vi "GEA2 FP ERDs.vi"(4 "2019 Inverter CMDs":T3[](array[typedef])=[{"ERD Number"=62218, "Data Type"=enum."string"}, {"ERD Number"=62229, "Data Type"=enum."string"}, {"ERD Number"=62224, "Data Type"=enum."string"}] {"ERD Number" format="%.0x"}, 6 "Inverter Address":T2={"Source"=240, "Destination"=63} {"Destination" format="%.0x"; "Source" format="%.0x"}, 8 "Error In":errorcluster, 10 "GEA2 Event Registration In":refnum<event-registration>, 11 ".NET Refnum in":refnum<k24>) -> (0 "Error Out":errorcluster, 1 "Data":string[][](array[string]), 2 "GEA2 Event Registration Out":refnum<event-registration>, 3 ".NET Refnum out":refnum<k24>, 5 "ERD Data Out":T1[](array[typedef]) {"ERD Number" format="%.0x"})   [LabVIEW 2016]
uses:
  type defs/ERD Read Data In.ctl
  type defs/Data Type.ctl
  type defs/Source_Destination.ctl
  C:/Technology Lab/NI-2010/Trunk/Utility/LabVIEW GEA2 Toolkit v1.0.0.0/Appliance.NET/GeaCommunication.dll
  Appliance.NET/GeaCommunication.dll
  type defs/Data Out.ctl
  type defs/ERD Read Data Out.ctl
  <vilib>/Utility/error.llb/whitespace.ctl
  library/GEA2_Toolkit.lvlib
panel:
  in  "#ERDs per message":i32=15
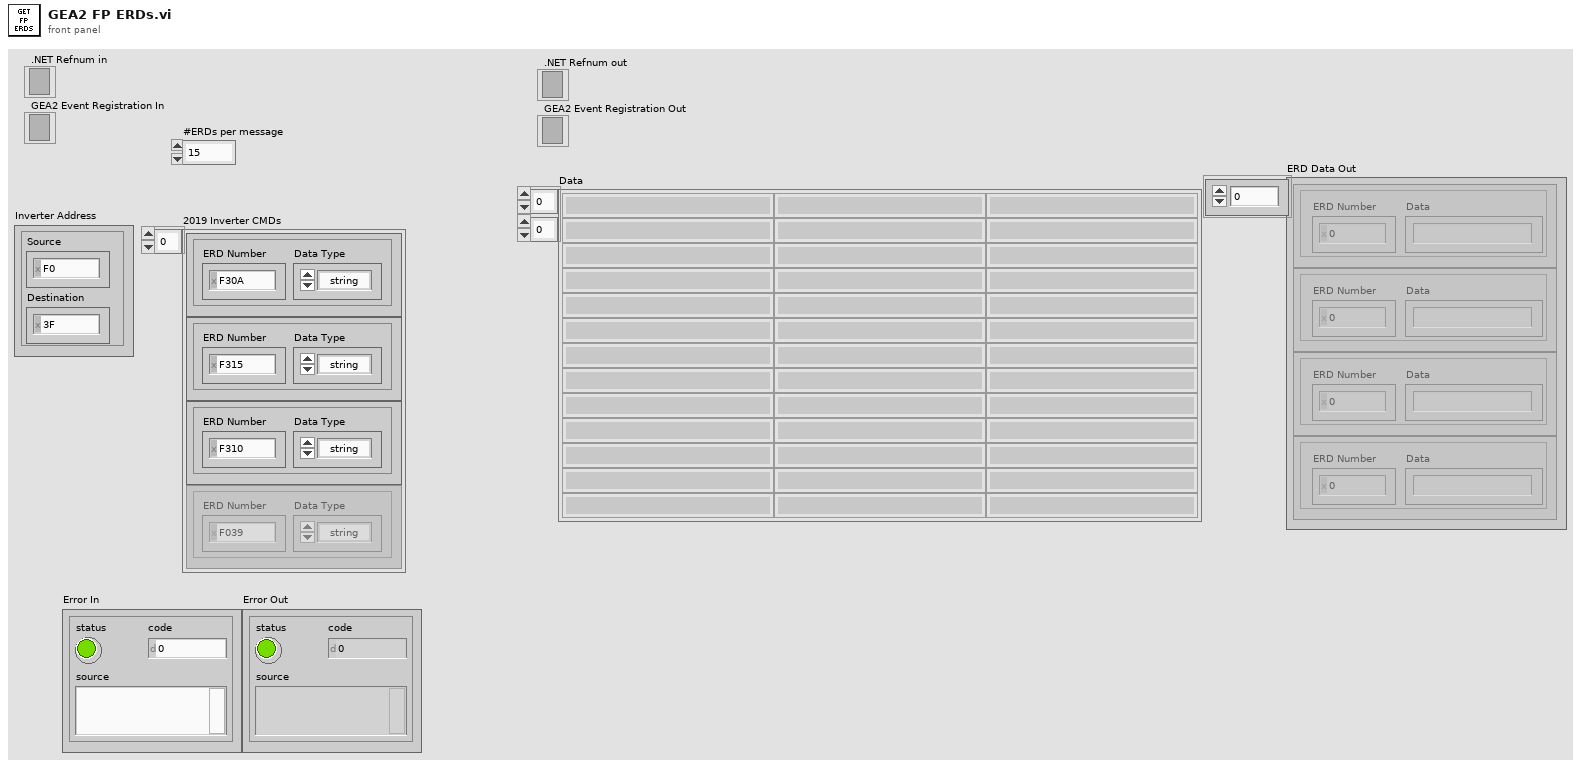
[diagram p1: front panel]
types:
  T1 = typedef "GEA2_Toolkit.lvlib/ERD Read Data Out.ctl" = cluster{"ERD Number":u16, "Data":string}
  T2 = typedef "GEA2_Toolkit.lvlib/Source_Destination.ctl" = cluster{"Source":u8, "Destination":u8}
  T3 = typedef "GEA2_Toolkit.lvlib/ERD Read Data In.ctl" = cluster{"ERD Number":u16, "Data Type":T4}
  T4 = typedef "GEA2_Toolkit.lvlib/Data Type.ctl" = enum16{"string", "boolean", "uint8_t", "uint16_t", "uint32_t", "uint64_t"}
  T5 = typedef "whitespace.ctl" = u16
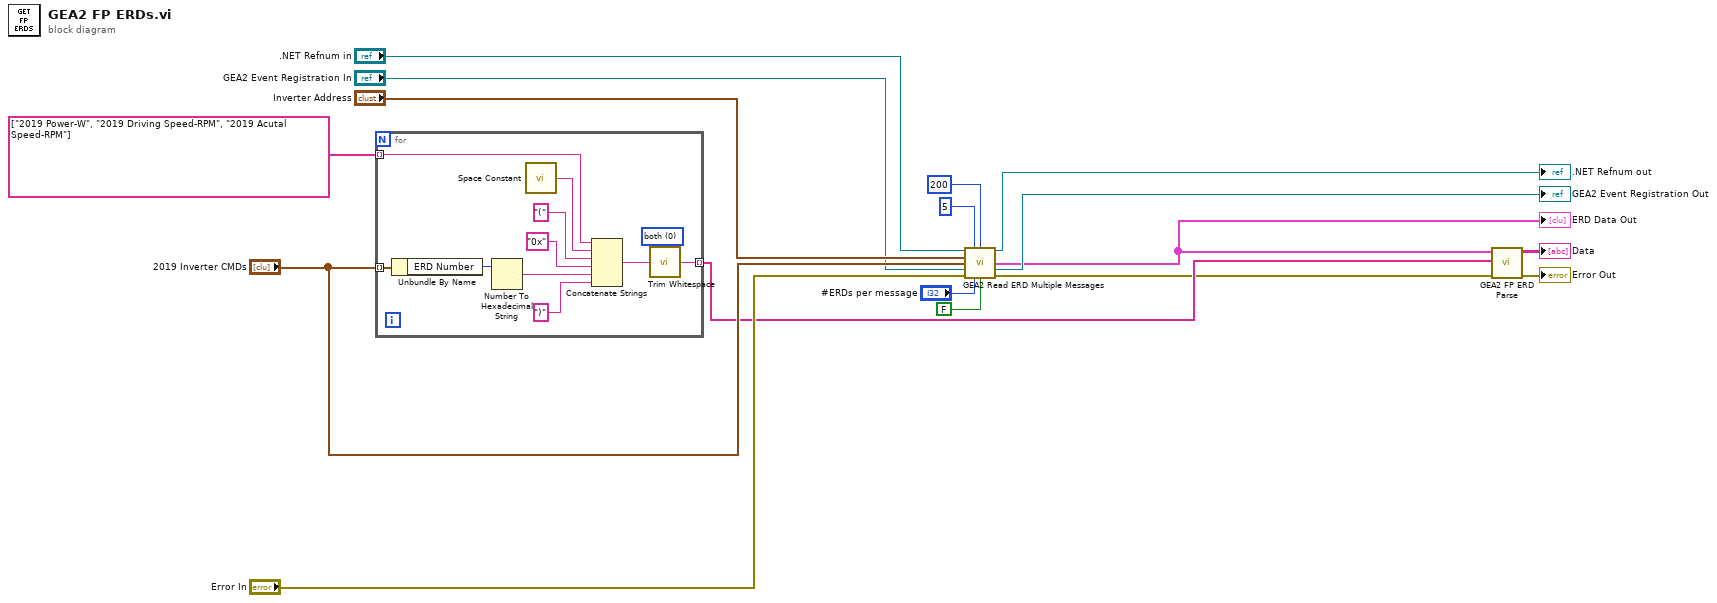
[diagram p0: block diagram]
diagram:
  n1 = for {
    tunnel: "2019 Inverter CMDs" -> [w28] mode=indexing
    tunnel: [w18] -> w4 mode=indexing
    tunnel: string[] ["2019 Power-W", "2019 Driving Speed-RPM", "2019 Acutal Speed-RPM"] -> [w21] mode=indexing
    w20 = T5 0 items=["both", "start of string", "end of string"] ("location (both)")
    n2 = Unbundle By Name(w28) -> ("ERD Number"=w27:u16)
    n3 = Number To Hexadecimal String(2:w27) -> (0:w26:string)  [unwired: 1 in]
    n4 = call <vilib>:"Space Constant.vi"() -> ("String"=w22:string)
    n5 = Concatenate Strings(w21, w22, "(" ("string"), "0x" ("string"), w26, ")" ("string")) -> (w19:string)
    n6 = call <vilib>:"Trim Whitespace.vi"("string"=w19, "location (both)"=w20) -> ("trimmed string"=w18:string)
  }
  n7 = call "GEA2 Read ERD Multiple Messages.vi"("GEA2 Reference In"=".NET Refnum in", "Retry Count"=5, "Read Timeout (ms)"=u32 200, "GEA Inputs"="Inverter Address", "Read ERD List"="2019 Inverter CMDs", "GEA2 Event Registration"="GEA2 Event Registration In", "Error In"="Error In", "#ERDs per message"="#ERDs per message", "Verify ERD Response?"=FALSE) -> ("GEA2 Reference Out"=→".NET Refnum out":refnum<k24>, "ERD Data Out"=w5:T1[], "Event Registration Refnum"=→"GEA2 Event Registration Out":refnum<event-registration>, "Error Out"=w2:errorcluster)  [unwired: 2 in, 1 out]
  "ERD Data Out" <- w5
  n8 = call "GEA2 FP ERD Parse.vi"("Error In"=w2, "Header"=w4, "ERD Data Out"=w5) -> ("Error Out"=→"Error Out":errorcluster, "Array out"=→"Data":string[][])  [unwired: 7 in]
